vi "Magnet Power Calc.vi"(0 "Current":dbl format="%.2f", 1 "Magnet Configuration Data":T1 {"Scale Factors" format="%.3f"; "Offsets" format="%.3f"; "Temp Coef" format="%.4g"; "Maximum Coil Currents" format="%.2g"; "Coil Inductances" format="%.3g"; "Pressure Range" format="%.2f"}) -> (2 "Magnet Voltage":dbl format="%.1f", 3 "Bus Voltage":dbl format="%.1g", 4 "Transistor Voltage":dbl=12.0, 5 "Power":dbl)   [LabVIEW 2019]
doc: "Takes the measured magnet parameters and resistive coefficients and calculates the expected voltages on the coils from the current and input water temperature. Also calculates the product of the current and the average temperature of each coil. The actual calculations are done in the sub VI \"Coil V to Temp\"\nScott Hannahs, NHMFL-FSU, April 1995"
uses:
  Sub Controls/RMPS Magnet Config.ctl
panel:
  # "kA"
  # "MW"
  # "Tin"
  # "Tout"
  # "Pin"
  # "Pout"
  # "I"
  # "WDTin"
  # "PSEnb"
  # "CellFLT"
  # "WDTout"
  # "BTFlt"
  # "BTvolt"
  # "Va"
  # "Vb"
  # "Vc"
  # "Vd"
  # "Tin"
  # "Tout"
  # "Pin"
  # "Pout"
  # "I"
  # "WDTin"
  # "PSEnb"
  # "CellFLT"
  # "WDTout"
  # "BTFlt"
  # "BTvolt"
  # "Va"
  # "Vb"
  # "Vc"
  # "Vd"
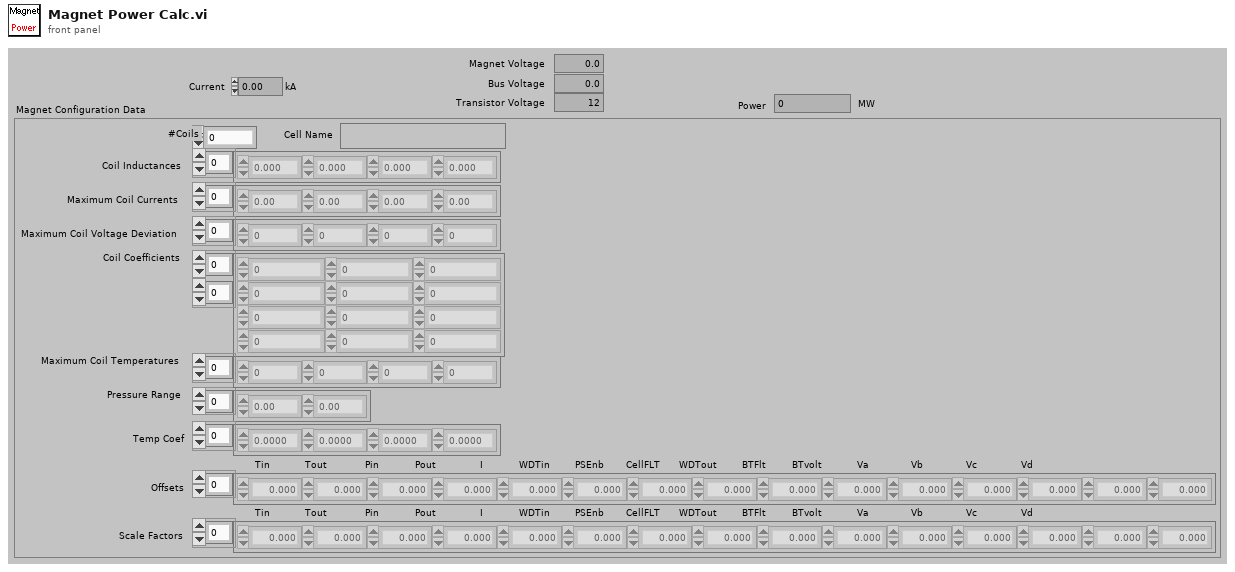
[diagram p1: front panel]
types:
  T1 = typedef "RMPS Magnet Config.ctl" = cluster{"#Coils":u32, "Coil Inductances":dbl[], "Maximum Coil Currents":dbl[], "Maximum Coil Voltage Deviation":dbl[], "Coil Coefficients":dbl[][], "Maximum Coil Temperatures":dbl[], " Pressure Range":dbl[], "Temp Coef":dbl[], "Offsets":dbl[], "Scale Factors":dbl[], "Cell Name":string}
  T2 = cluster{"Coil Coefficients":dbl[][], "Temp Coef":dbl[]}
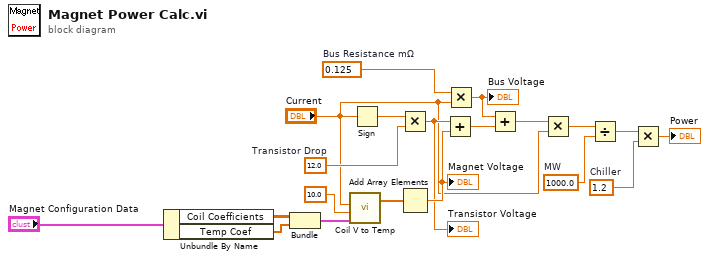
[diagram p0: block diagram]
diagram:
  w5 = 0.125  # Bus Resistance mΩ
  w9 = 1.2  # Chiller
  w11 = 12.0  # Transistor Drop
  w15 = 1000.0  # MW
  n1 = Unbundle By Name("Magnet Configuration Data") -> ("Coil Coefficients"=w20:dbl[][], "Temp Coef"=w19:dbl[])
  n2 = Bundle("Coil Coefficients"=w20, "Temp Coef"=w19) -> (w18:T2)  [unwired: 1 in]
  n3 = call "Coil V to Temp.vi"("Coil Specs"=w18, "T inlet"=10.0 ("Temp"), "I"="Current") -> ("Expected Voltage"=w13:dbl[])  [unwired: 1 in, 1 out]
  n4 = Sign(1:"Current") -> (0:w2:dbl)
  n5 = Multiply(x=w2, y=w11) -> (x*y=w4:dbl)
  "Transistor Voltage" <- w4
  n6 = Add Array Elements(numeric array=w13) -> (sum=w17:dbl)
  "Magnet Voltage" <- w17
  n7 = Add(x=w4, y=w17) -> (x+y=w12:dbl)
  n8 = Multiply(x=w5, y="Current") -> (x*y=w6:dbl)
  "Bus Voltage" <- w6
  n9 = Add(x=w6, y=w12) -> (x+y=w7:dbl)
  n10 = Multiply(x=w7, y="Current") -> (x*y=w8:dbl)
  n11 = Divide(x=w8, y=w15) -> (x/y=w16:dbl)
  n12 = Multiply(x=w16, y=w9) -> (x*y=→"Power":dbl)
